vi "Vision Processing.vi"(4 "error in (no error)":errorcluster) -> ()   [LabVIEW 2012]
doc: "This VI runs in parallel to other tasks. It gets images from the camera, processes them for color or shape and use that information to affect robot behavior."
uses:
  Robot Global Data.vi
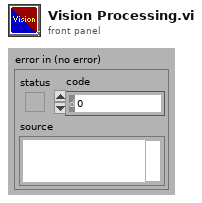
[diagram p1: front panel]
types:
  T1 = typedef "Image Type" = u32
  T2 = typedef "WPI_CameraDevRef.ctl" = cluster{"Camera Address":string, "CameraStatus":errorcluster, "Acquire Image Notifier":refnum<notifier>}
  T3 = typedef "IMAQ Image.ctl" = refnum<image>
  T4 = typedef "WPI_CameraImageSize.ctl" = enum16{"640x480", "320x240", "160x120"}
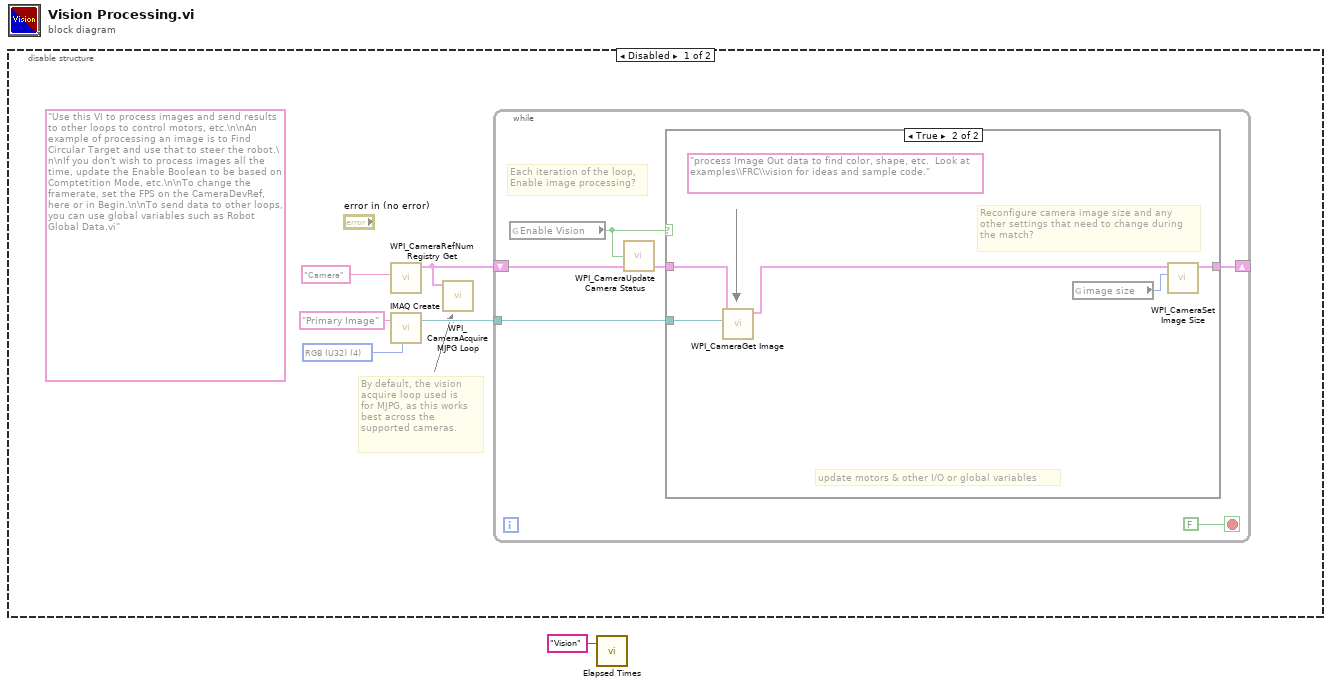
[diagram p0: block diagram]
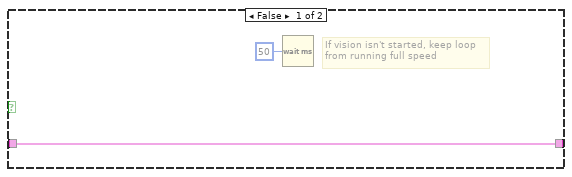
[diagram p2: hidden frame]
diagram:
  n1 = disable-structure shown="Disabled" {
    frame Disabled {
      (unwired) "Use this VI to process images and send results to other loops to control motors, etc.\n\nAn example of processing an image is to Find Circular Target and use that to steer the robot.\n\nIf you don't wish to process images all the time, update the Enable Boolean to be based on Comptetition Mode, etc.\n\nTo change the framerate, set the FPS on the CameraDevRef, here or in Begin.\n\nTo send data to other loops, you can use global variables such as Robot Global Data.vi"
      w6 = T1 4 items=["Grayscale (U8)", "Grayscale (I16)", "Grayscale (SGL)", "Complex (CSG)", "RGB (U32)", "HSL (U32)", "RGB (U64)"] ("Image Type")
      # "By default, the vision\nacquire loop used is\nfor MJPG, as this works\nbest across the\nsupported cameras."
      n2 = call <vilib>:"WPI_CameraRefNum Registry Get.vi"("refnum name"="Camera") -> ("CameraDevRef"=w2:T2)  [unwired: 1 in, 9 out]
      n3 = call "IMAQ Create"("Image Name"="Primary Image", "Image Type"=w6) -> ("New Image"=w4:T3)  [unwired: 2 in, 2 out]
      n4 = call <vilib>:"WPI_CameraAcquire MJPG Loop.vi"("CameraDevRef"=w2) -> ()  [unwired: 11 in]
      n5 = while {
        shift-right: [w11] -> _
        shift-left: w2 -> [w9]
        tunnel: w4 -> [w10]
        stop <- FALSE stop-if-true
        # "Each iteration of the loop,\nEnable image processing?"
        n6 = global read "Robot Global Data.vi" "Enable Vision"() -> (w7:bool)
        n7 = call <vilib>:"WPI_CameraUpdate Camera Status.vi"("CameraDevRef In"=w9, "Enable Vision"=w7) -> ("CameraDevRef Out"=w8:T2)  [unwired: 3 in]
        n8 = case shown="True" w7 {
          tunnel: w10 -> [_ w18]
          tunnel: [w14 w19] -> w11
          tunnel: w8 -> [w14 w16]
          frame False {
            # "If vision isn't started, keep loop\nfrom running full speed"
            n9 = Wait (ms)(milliseconds to wait=u32 50) -> ()  [unwired: 1 out]
          }
          frame True {
            (unwired) "process Image Out data to find color, shape, etc.  Look at examples\\FRC\\vision for ideas and sample code."
            # "update motors & other I/O or global variables"
            # "Reconfigure camera image size and any\nother settings that need to change during\nthe match?"
            n10 = call <vilib>:"WPI_CameraGet Image.vi"("Image"=w18, "CameraDevRef"=w16) -> ("CameraDevRef Out"=w15:T2)  [unwired: 1 in, 8 out]
            n11 = global read "Robot Global Data.vi" "image size"() -> (w17:T4)
            n12 = call <vilib>:"WPI_CameraSet Image Size.vi"("Image Size"=w17, "CameraDevRef"=w15) -> ("CameraDevRef Out"=w19:T2)  [unwired: 1 in, 8 out]
          }
        }
      }
    }
    frame Enabled {
    }
  }
  n13 = call "Elapsed Times.vi"("Call Name"="Vision") -> ()  [unwired: 2 in, 1 out]
